vi "Set Server State.vi"(8 "error in (no error)":errorcluster, 10 "New State":T1, 11 "OOP Query Server in":refnum<class "OOP Query Server.lvclass">) -> (0 "error out":errorcluster, 2 "Previous State":T1, 3 "OOP Query Server out":refnum<class "OOP Query Server.lvclass">)   [LabVIEW 2019, in "OOP Query Server.lvlib" / "OOP Query Server.lvclass"]
uses:
  OOP Query Server.lvclass
  typeDefs/Server State Data.ctl
  OOP Query Server.lvclass/OOP Query Server.ctl
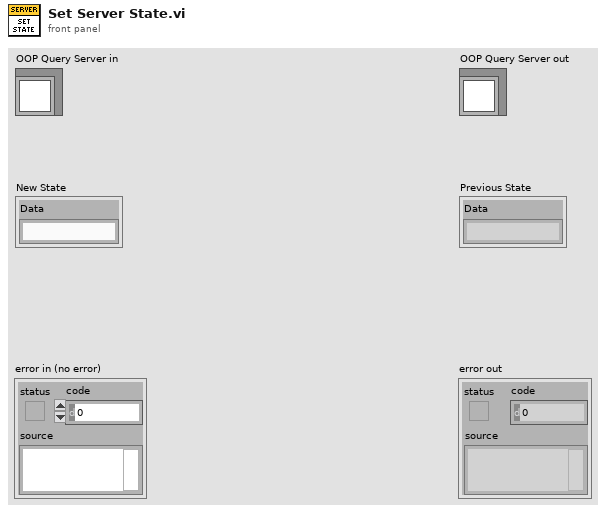
[diagram p1: front panel]
types:
  T1 = typedef "OOP Query Server.lvlib/OOP Query Server.lvclass/Server State Data.ctl" = cluster{"Data":string}
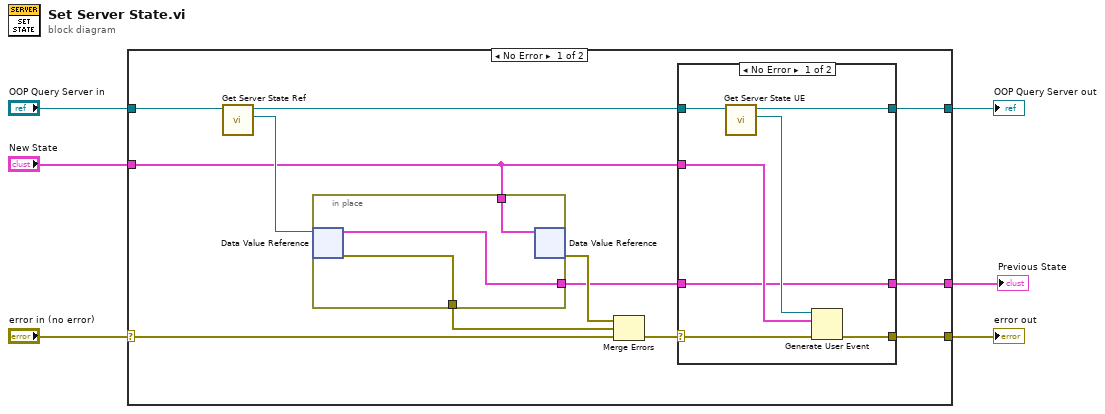
[diagram p0: block diagram]
diagram:
  n1 = case shown="No Error" "error in (no error)" {
    selector: "error in (no error)" -> [w14 w34]
    tunnel: [w11 w34] -> w5
    tunnel: [w10 w33] -> w3
    tunnel: "OOP Query Server in" -> [w18 w33]
    tunnel: "New State" -> [w9 w32]
    tunnel: [w7 w32] -> w1
    frame No Error {
      n2 = call "Get Server State Ref.vi"("OOP Query Server in"=w18) -> ("Server State Ref"=w17:refnum<data-value>, "OOP Query Server out"=w13:refnum<class "OOP Query Server.lvclass">)  [unwired: 9 in]
      n3 = in-place {
        in-place-border: w9 -> [w31]
        in-place-border: [w30] -> w8
        in-place-border: [w29] -> w15
        n4 = in-place-dvr #1(w17) -> (w30:T1, w29:errorcluster)
        n5 = in-place-dvr #1(w31) -> (w16:errorcluster)  [unwired: 1 out]
      }
      n6 = Merge Errors(w16, w15, w14) -> (w12:errorcluster)
      n7 = case shown="No Error" w12 {
        selector: w12 -> [w24 w28]
        tunnel: w13 -> [w25 w27]
        tunnel: [w23 w28] -> w11
        tunnel: [w21 w27] -> w10
        tunnel: w9 -> [w20 _]
        tunnel: w8 -> [w19 w26]
        tunnel: [w19 w26] -> w7
        frame No Error {
          n8 = call "Get Server State UE.vi"("OOP Query Server in"=w25) -> ("Server Internal State UE"=w22:refnum<user-event>, "OOP Query Server out"=w21:refnum<class "OOP Query Server.lvclass">)  [unwired: 9 in]
          n9 = Generate User Event(user event=w22, event data cluster=w20, error in=w24) -> (error out=w23:errorcluster)  [unwired: 1 in, 1 out]
        }
        frame Error {
        }
      }
    }
    frame Error {
    }
  }
  "error out" <- w5
  "OOP Query Server out" <- w3
  "Previous State" <- w1
